vi "Cleanup.vi"(8 "error in (no error)":errorcluster, 11 "TCP Client in":refnum<class "TCP Client.lvclass">) -> (0 "error out":errorcluster)   [LabVIEW 2024, in "Stream-TCP.lvlib" / "TCP Client.lvclass"]
uses:
  TCP Client.lvclass
  TCP Client.lvclass/TCP Client.ctl
  lv-stream/stream/Connection/Connection.lvclass
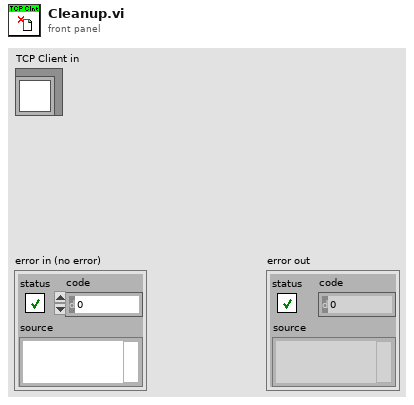
[diagram p1: front panel]
types:
  T1 = typedef "Stream-TCP.lvlib/Client Command Queue.ctl" = refnum<queue>
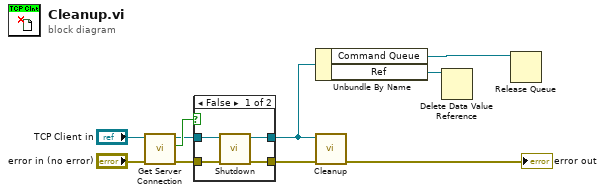
[diagram p0: block diagram]
diagram:
  n1 = call "Get Server Connection.vi"("error in (no error)"="error in (no error)", "TCP Client in"="TCP Client in") -> ("error out"=w1:errorcluster, "Is Server Connection"=w3:bool, "TCP Client out"=w2:refnum<class "TCP Client.lvclass">)  [unwired: 7 in]
  n2 = case shown="False" w3 {
    tunnel: [w14 w15] -> w7
    tunnel: [w13 w16] -> w6
    tunnel: w2 -> [w12 w16]
    tunnel: w1 -> [w11 w15]
    frame False {
      n3 = call "Shutdown.vi"("error in (no error)"=w11, "TCP Client in"=w12) -> ("error out"=w14:errorcluster, "TCP Client out"=w13:refnum<class "TCP Client.lvclass">)  [unwired: 8 in]
    }
    frame True {
    }
  }
  n4 = Unbundle By Name(w6) -> ("Command Queue"=w9:T1, "Ref"=w10:refnum<data-value>)
  n5 = call-parent "Cleanup.vi"("error in (no error)"=w7, "Connection in"=w6) -> ("error out"=→"error out":errorcluster)  [unwired: 9 in]
  n6 = Delete Data Value Reference(data value reference=w10) -> ()  [unwired: 1 in, 2 out]
  n7 = Release Queue(queue=w9) -> ()  [unwired: 2 in, 3 out]
